vi "lab_3_forloop.vi"() -> ()   [LabVIEW 2015]
panel:
  in  "milliseconds to wait":u32=1
  out "Last iteration":dbl=9.0
  out "Waveform Graph":i32[](graph)=[0, 1, 2, 3, 4, 5, 6, 7, 8, 9]
  out "current iteration":dbl=9.0
  in  "Numer of iterations":i32=10
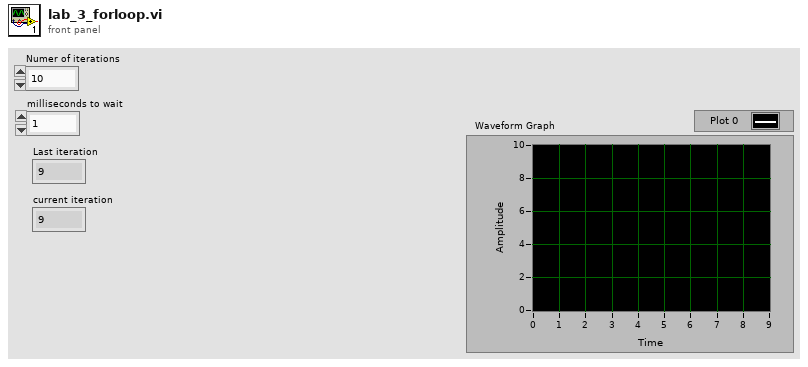
[diagram p1: front panel]
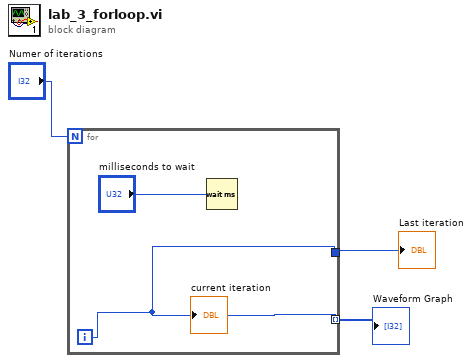
[diagram p0: block diagram]
diagram:
  n1 = for {
    N: "Numer of iterations" -> [_]
    tunnel: [w5] -> w2 mode=indexing
    tunnel: [w5] -> w1
    i -> [w5]
    n2 = Wait (ms)(milliseconds to wait="milliseconds to wait") -> ()  [unwired: 1 out]
    "current iteration" <- w5
  }
  "Waveform Graph" <- w2
  "Last iteration" <- w1
